vi "detElementNameWithAttributes.vi"(8 "error in (no error)":errorcluster, 10 "XML In":string, 11 "Element in":refnum<class "XMLParser.lvclass">) -> (0 "error out":errorcluster, 2 "ElementName":string, 3 "Element out":refnum<class "XMLParser.lvclass">)   [LabVIEW 2016, in "XML.lvlib" / "XMLParser.lvclass"]
doc: "This method determines element name if there are attributes in the current element."
uses:
  <userlib>/Common/XML/XMLParser/XMLParser.lvclass
  <userlib>/Common/XML/XMLParser/XMLParser.lvclass/XMLParser.ctl
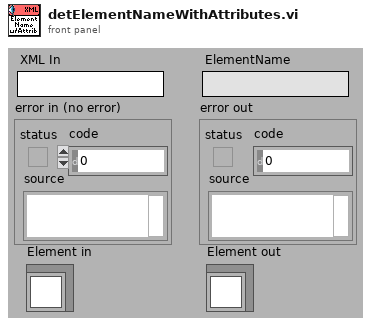
[diagram p1: front panel]
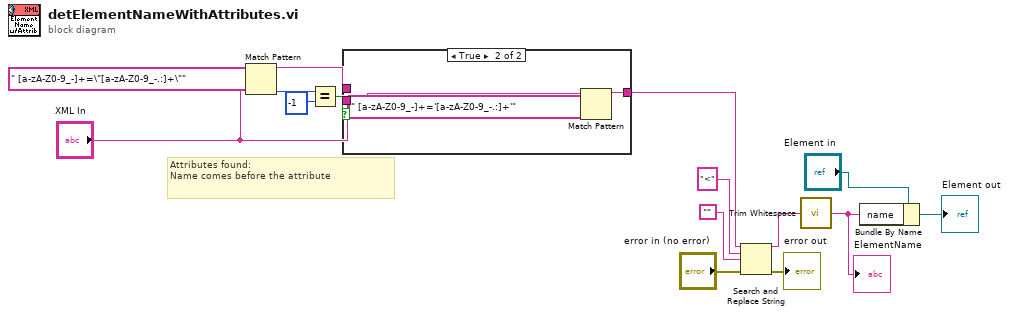
[diagram p0: block diagram]
diagram:
  # "Attributes found:\nName comes before the attribute"
  n1 = Match Pattern(string="XML In", regular expression=" [a-zA-Z0-9_-]+=\"[a-zA-Z0-9_-.:]+\"") -> (before substring=w2:string, offset past match=w7:i32)  [unwired: 1 in, 2 out]
  n2 = Equal?(x=w7, y=-1) -> (x = y?=w5:bool)
  n3 = case shown="True" w5 {
    tunnel: "XML In" -> [_ w18]
    tunnel: [w16 w17] -> w3
    tunnel: w2 -> [w16 _]
    frame False {
    }
    frame True {
      n4 = Match Pattern(string=w18, regular expression=" [a-zA-Z0-9_-]+='[a-zA-Z0-9_-.:]+'") -> (before substring=w17:string)  [unwired: 1 in, 3 out]
    }
  }
  n5 = Search and Replace String(input string=w3, search string="<", replace string="", error in="error in (no error)") -> (result string=w10:string, error out=→"error out":errorcluster)  [unwired: 4 in, 2 out]
  n6 = call <vilib>:"Trim Whitespace.vi"("string"=w10) -> ("trimmed string"=w9:string)  [unwired: 1 in]
  "ElementName" <- w9
  n7 = Bundle By Name(cluster="Element in", "name"=w9) -> (→"Element out":refnum<class "XMLParser.lvclass">)
